vi "IndexDatabaseData.vi"(10 "index":i32, 11 "recordset data":variant[](array[variant])) -> (3 "数组":string[](array[string]))   [LabVIEW 2014, in "DataBase.lvlib"]
uses:
  DataBase.lvlib
  <vilib>/addons/database/_DB Variant To Data/Database Variant To Data.xnode
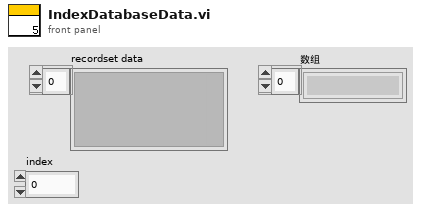
[diagram p1: front panel]
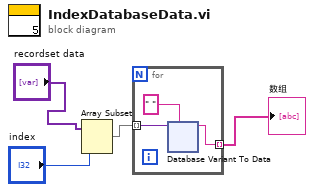
[diagram p0: block diagram]
diagram:
  n1 = Array Subset(array="recordset data", index="index") -> (w3:variant[])  [unwired: 1 in]
  n2 = for {
    tunnel: w3 -> [w5] mode=indexing
    tunnel: [w6] -> w4 mode=indexing
    n3 = xnode "Database Variant To Data"("database variant"=w5, "type"=" ") -> ("data"=w6:string)  [unwired: 1 in, 1 out]
  }
  "数组" <- w4
